vi "Get Value (from Key).vi"(8 "error in (no error)":errorcluster, 10 "key":string, 11 "URI-Component.Query in":refnum<class "URI-Component.Query.lvclass">) -> (0 "error out":errorcluster, 1 "value":string, 2 "key dup":string, 3 "URI-Component.Query":refnum<class "URI-Component.Query.lvclass">, 4 "found":bool)   [LabVIEW 2013, in "openURI.lvlib" / "URI-Component.Query.lvclass"]
uses:
  URI-Component.Query.lvclass
  URI-Component.Query.lvclass/URI-Component.Query.ctl
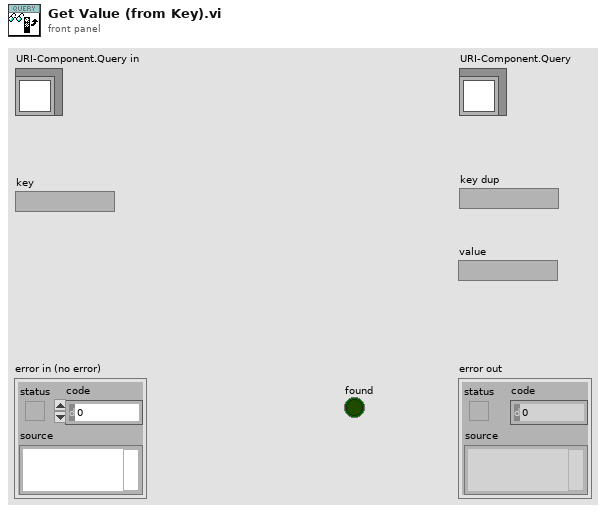
[diagram p1: front panel]
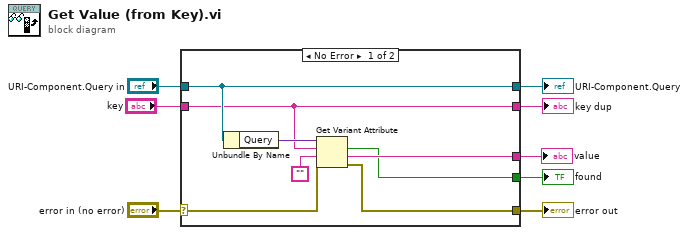
[diagram p0: block diagram]
diagram:
  n1 = case shown="No Error" "error in (no error)" {
    selector: "error in (no error)" -> [w10 w18]
    tunnel: [w9 w18] -> w7
    tunnel: [w16 w19] -> w5
    tunnel: "URI-Component.Query in" -> [w16 w19]
    tunnel: [w14 w17] -> w4
    tunnel: "key" -> [w14 w17]
    tunnel: [w12 _] -> w2
    tunnel: [w11 _] -> w1
    frame No Error {
      n2 = Unbundle By Name(w16) -> ("Query"=w15:variant)
      n3 = Get Variant Attribute(Variant=w15, name=w14, default value (empty Variant)="", error in=w10) -> (found=w11:bool, value=w12:string, error out=w9:errorcluster)  [unwired: 1 out]
    }
    frame Error {
    }
  }
  "error out" <- w7
  "URI-Component.Query" <- w5
  "key dup" <- w4
  "value" <- w2
  "found" <- w1
